vi "Magnet Configure (Poly).vi"   [LabVIEW 2016, in "Hall Effect Library.lvlib"]
uses:
  Hall Effect Library.lvlib
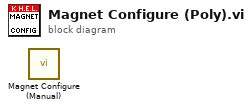
[diagram p0: block diagram]
diagram:
  n1 = call "Magnet Configure (Manual).vi"() -> ()  [unwired: 10 in, 2 out]
